vi "get control.vi"(8 "error in (no error)":errorcluster, 11 "path":string) -> (0 "error out":errorcluster, 3 "control_frontpanel_image":picture)   [LabVIEW 2020]
doc: "Returns a screenshot of the content (frontpanel) of a .ctl file. Use this to understand the content of a LabVIEW type definition or custom control."
uses:
  G-AI Core/G-AI Core.lvlib
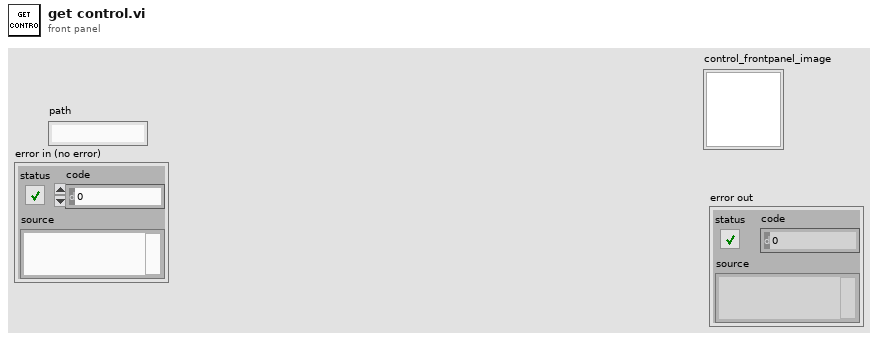
[diagram p1: front panel]
types:
  T1 = typedef "imagedata.ctl" = cluster{"image type":i32, "image depth":i32, "image":u8[], "mask":u8[], "colors":u32[], "Rectangle":cluster{"left":i16, "top":i16, "right":i16, "bottom":i16}}
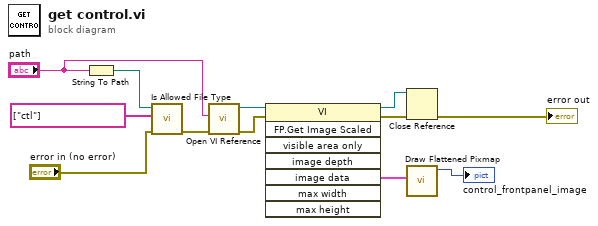
[diagram p0: block diagram]
diagram:
  n1 = String To Path(string="path") -> (path=w4:path)
  n2 = call "Is Allowed File Type.vi"("error in (no error)"="error in (no error)", "y"=string[] ["ctl"], "Path"=w4) -> ("error out"=w3:errorcluster)  [unwired: 8 in]
  n3 = call "Open VI Reference.vi"("error in"=w3, "VI Path"="path") -> ("error out"=w10:errorcluster, "VI Refnum"=w11:refnum<vi>)  [unwired: 8 in]
  n4 = invoke class="VI" method="FP.Get Image Scaled"(reference=w11, error in=w10) -> (reference out=w8:refnum<vi>, error out=w9:errorcluster, "image data"=w12:T1)  [unwired: 6 in, 5 out]
  n5 = Close Reference(reference=w8, error in (no error)=w9) -> (error out=→"error out":errorcluster)
  n6 = call <vilib>:"Draw Flattened Pixmap.vi"("image data"=w12) -> ("new picture"=→"control_frontpanel_image":picture)  [unwired: 8 in]
